vi "beamSplitterVI.vi"() -> ()   [LabVIEW 2013]
panel:
  out "Reflected Pulses":dbl[][](array[numeric])
  out "Transmit Pulses":dbl[][](array[numeric])
  in  "Input Pulse":dbl[][](array[numeric])
  in  "Transmit %":dbl
  # "frequency[Hz], amplitude[V], delay [s], polarization[0,1], power[fraction]"
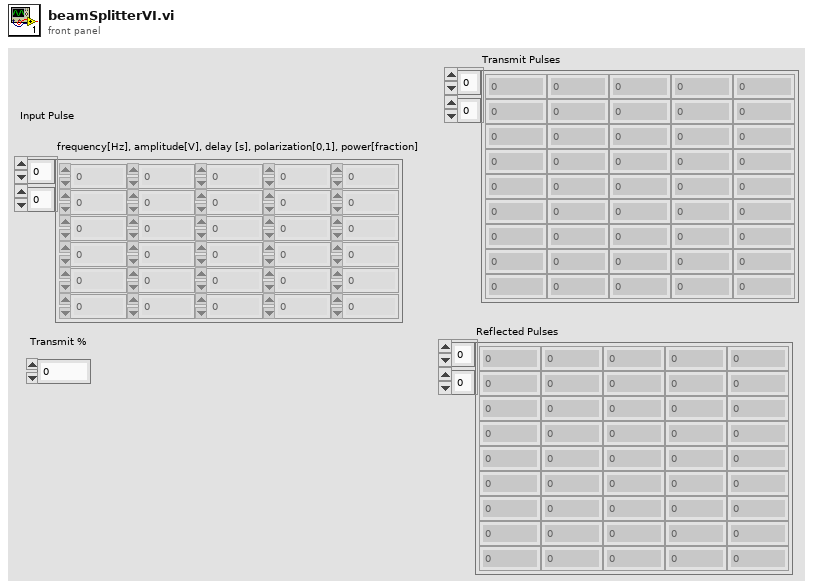
[diagram p1: front panel]
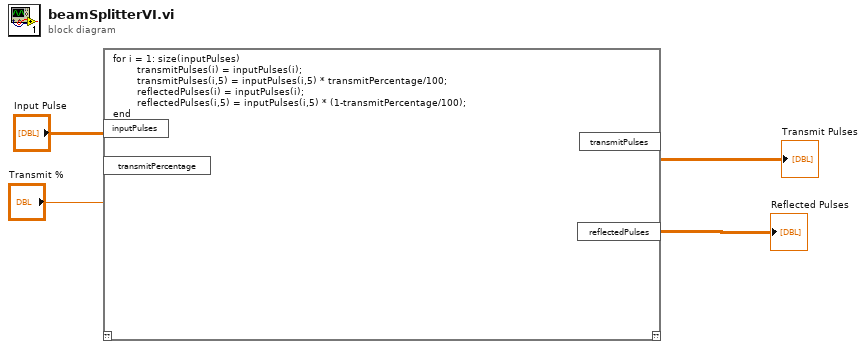
[diagram p0: block diagram]
diagram:
  n1 = script code="for i = 1: size(inputPulses)\n        transmitPulses(i) = inputPulses(i);\n        transmitPulses(i,5) = inputPulses(i,5) * transmitPercentage/100;\n        reflectedPulses(i) = inputPulses(i);\n        reflectedPulses(i,5) = inputPulses(i,5) * (1-transmitPercentage/100);\nend"("inputPulses"="Input Pulse", "transmitPercentage"="Transmit %") -> ("transmitPulses"=→"Transmit Pulses":dbl[][], "reflectedPulses"=→"Reflected Pulses":dbl[][])  [unwired: 1 in, 1 out]
